vi "CVCPdll.vi"(8 "error in (no error)":errorcluster, 9 "z":dbl[](array[numeric]), 10 "D":dbl, 11 "t":dbl) -> (0 "error out":errorcluster, 2 "Cv":dbl, 3 "Cp":dbl)   [LabVIEW 2016]
doc: "subroutine CVCP (t,D,z,cv,cp)\n\nCompute isochoric (constant volume) and isobaric (constant pressure)\nheat capacity as functions of temperature, density, and composition\nusing core functions\n\nBased on derivations in Younglove & McLinden, JPCRD 23 #5, 1994,\nequation A15, A16\n\nINPUTS:\nt -- temperature [K]\nD -- molar density [mol/L]\nz -- composition [array of mol frac]\n\nOUTPUTS:\ncv -- isochoric heat capacity [J/mol-K]\ncp -- isobaric heat capacity [J/mol-K]"
uses:
  REFPROP.DLL
panel:
  # "REFPROP-CVCdll.vi"
  # "void  CVCPdll(double *t, double *D, double *z, double *cv, double *cp)"
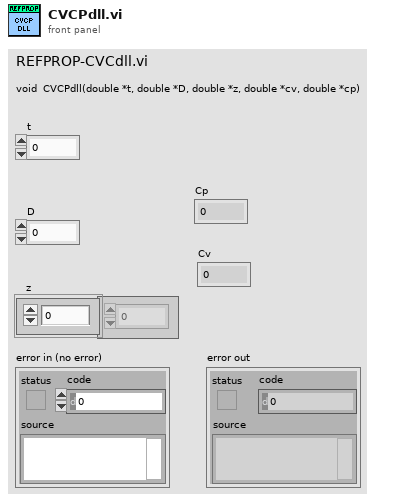
[diagram p1: front panel]
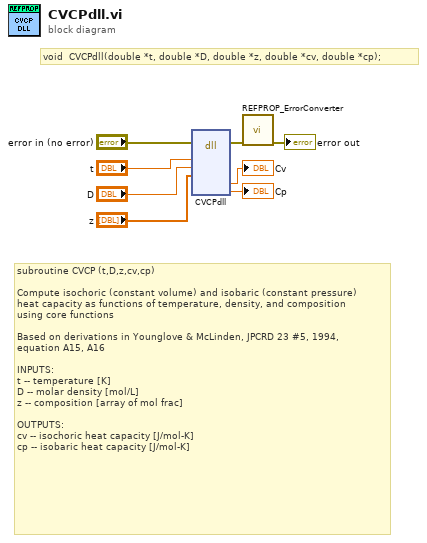
[diagram p0: block diagram]
diagram:
  # "void  CVCPdll(double *t, double *D, double *z, double *cv, double *cp);"
  # "subroutine CVCP (t,D,z,cv,cp)\n\nCompute isochoric (constant volume) and isobaric (constant pressure)\nheat capacity as functions of temperature, density, and composition\nusing core functions\n\nBased on derivations in Younglove & McLinden, JPCRD 23 #5, 1994,\nequation A15, A16\n\nINPUTS:\nt -- temperature [K]\nD -- molar density [mol/L]\nz -- composition [array of mol frac]\n\nOUTPUTS:\ncv -- isochoric heat capacity [J/mol-K]\ncp -- isobaric heat capacity [J/mol-K]"
  n1 = dll-call lib="S:/009 - Testing/02 - Performance Testing/REFPROP/REFPROP.*" fn="CVCPdll"(error in="error in (no error)", "t"="t", "D"="D", "z"="z") -> (error out=w3:errorcluster, "cv"=→"Cv":dbl, "cp"=→"Cp":dbl)  [unwired: 8 in, 1 out]
  n2 = call "REFPROP_ErrorConverter.vi"("error in (no error)"=w3) -> ("error out"=→"error out":errorcluster)  [unwired: 10 in]
